vi "Acquire Data.vi"(6 "MemberAttendance":refnum<class "MemberAttendance.lvclass">, 8 "error in (no error)":errorcluster, 9 "ExcuseNotesHandler":refnum<class "ExcuseNotesHandler.lvclass">, 10 "TimeTable":refnum<class "TimeTable.lvclass">, 11 "AttendRecord.lvclass":refnum<class "AttendRecord.lvclass">) -> (0 "error out":errorcluster, 3 "AttendRecord.lvclass":refnum<class "AttendRecord.lvclass">)   [LabVIEW 2015]
uses:
  Member_Actor/MemberTable/TimeTable.lvclass
  MemberAttendance/MemberAttendance.lvclass
  ExcuseNotes/ExcuseNotesHandler.lvclass
  AttendRecord.lvclass
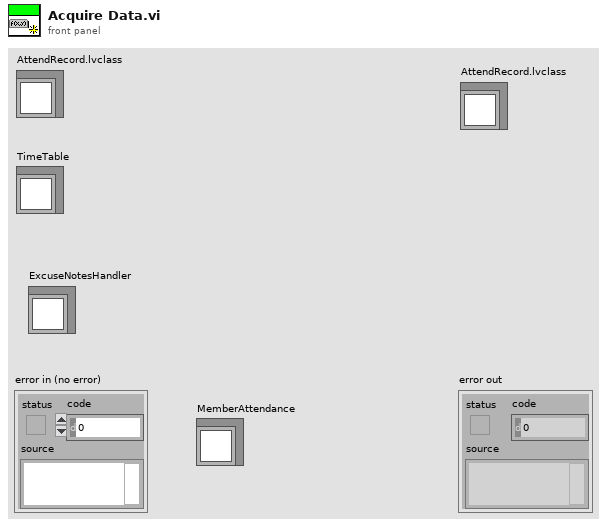
[diagram p1: front panel]
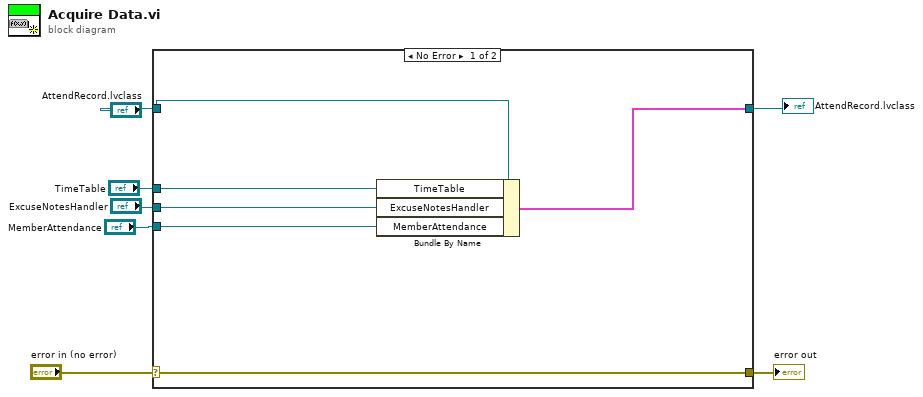
[diagram p0: block diagram]
diagram:
  n1 = case shown="No Error" "error in (no error)" {
    selector: "error in (no error)" -> [w13 w15]
    tunnel: [w13 w15] -> w6
    tunnel: [w11 w14] -> w1
    tunnel: "AttendRecord.lvclass" -> [w12 w14]
    tunnel: "TimeTable" -> [w10 _]
    tunnel: "ExcuseNotesHandler" -> [w9 _]
    tunnel: "MemberAttendance" -> [w8 _]
    frame No Error {
      n2 = Bundle By Name(cluster=w12, "TimeTable"=w10, "ExcuseNotesHandler"=w9, "MemberAttendance"=w8) -> (w11:cluster{})
    }
    frame Error {
    }
  }
  "error out" <- w6
  "AttendRecord.lvclass" <- w1
